vi "PV ActiveLine - Save Parameters.vi"(7 "W/R":bool, 8 "Fehler (Eingang)":errorcluster, 9 "use file number":i8=1 min=1 max=99 format="%02.0f", 10 "Setup parameters mode":i8(ring)=1 items=["save"=1, "restore"=2, "format"=3, "clear"=4], 11 "Referenz in":refnum<visa-resource-name>) -> (0 "Cluster (Ausgang)":errorcluster, 1 "Read Status":u16(ring) items=["Read Failed", "Read Ok"], 2 "Setup control mode OUT":i8(ring) items=["done / ready", "saving", "restoring", "formating", "clearing"], 3 "Referenz out":refnum<visa-resource-name>)   [LabVIEW 2013, in "PV ActiveLine.lvlib"]
doc: "SCM - Save Parameters\n\nTransmit: SCM [,a,bb]\nReceive: a\n\nSetup parameters,\na =\n0 –> Saving completed\n1 –> CSV file is being saved\n2 –> Loading all parameters from the USB memory stick onto the TPG 36x\n3 –> Formatting USB memory stick (FAT32)\n4 –> Deleting parameter files (ending CSV) from the USB memory stick\n\nbb = Number in the file name (0 … 99)\n\nGroup Setup\nThe group is only available when a USB memory stick formatted for the the FAT file system (FAT32) is plugged in. Use a max. 32 GB memory stick."
uses:
  <instrlib>/PV ActiveLine/PV ActiveLine.lvlib
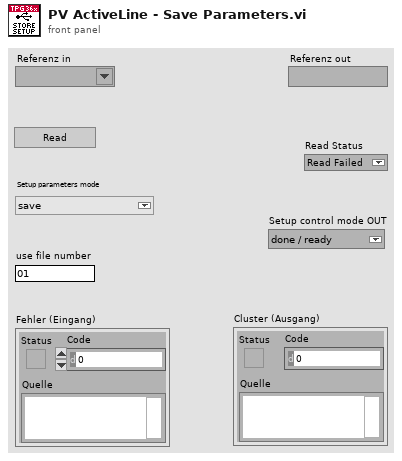
[diagram p1: front panel]
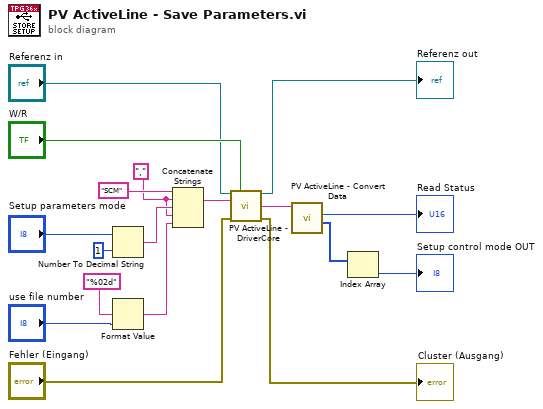
[diagram p0: block diagram]
diagram:
  w10 = "," ("Command")
  n1 = Number To Decimal String(number="Setup parameters mode", width (-)=i16 1) -> (decimal integer string=w15:string)
  n2 = Format Value(format string="%02d", value (0)="use file number") -> (output string=w7:string)  [unwired: 1 in]
  n3 = Concatenate Strings("SCM" ("Command"), w10, w15, w10, w7) -> (w13:string)
  n4 = call <instrlib>:"PV ActiveLine - DriverCore.vi"("Referenz in"="Referenz in", "Write/Read"="W/R", "Command"=w13, "Fehler (Eingang)"="Fehler (Eingang)") -> ("Referenz out"=→"Referenz out":refnum<visa-resource-name>, "String Out"=w4:string, "Cluster (Ausgang)"=→"Cluster (Ausgang)":errorcluster)  [unwired: 9 in]
  n5 = call <instrlib>:"PV ActiveLine - Convert Data.vi"("String in"=w4) -> ("Integer Out"=w2:i32[], "Read Status"=→"Read Status":u16)  [unwired: 7 in, 2 out]
  n6 = Index Array(array=w2) -> (element=→"Setup control mode OUT":i32)  [unwired: 1 in]
